vi "SingleElementsArray To Data_csm.vi"(7 "Pototype":variant, 8 "error in (no error)":errorcluster, 11 "DataElementArray":variant[](array[variant])) -> (0 "error out":errorcluster, 3 "Cluster":variant)   [LabVIEW 2017, in "API String Arguments Support.lvlib"]
doc: "This VI converts a DataELementArray to a Cluster."
uses:
  API String Arguments Support.lvlib
  <userlib>/_NEVSTOP/Communicable State Machine(CSM)/Communicable State Machine.lvlib
  <vilib>/Utility/Data Type/NI_Data Type.lvlib
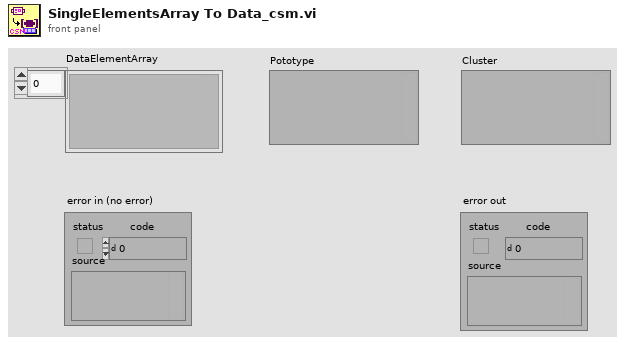
[diagram p1: front panel]
types:
  T1 = enum8{"<Null>", "I8", "I16", "I32", "I64", "U8", "U16", "U32", "U64", "SGL", "DBL", "EXT", "CSG", "CDB", "CXT", "0x0F", "0x10", "0x11", "0x12", "0x13", "0x14", "Enum U8", "Enum U16", "Enum U32", "Enum U64", "SGL PQ", "DBL PQ", "EXT PQ", "CSG PQ", "CDB PQ", "CXT PQ", "0x1F", "0x20", "Boolean", "0x22", "0x23", "0x24", "0x25", "0x26", "0x27", "0x28", "0x29", "0x2A", "0x2B", "0x2C", "0x2D", "0x2E", "0x2F", "String", "0x31", "Path", "Pict", "0x34", "0x35", "0x36", "DAQ", "0x38", "0x39", "0x3A", "0x3B", "0x3C", "0x3D", "0x3E", "0x3F", "Array", "0x41", "0x42", "0x43", "0x44", "0x45", "0x46", "0x47", "0x48", "0x49", "0x4A", "0x4B", "0x4C", "0x4D", "0x4E", "0x4F", "Cluster", "0x51", "0x52", "Variant", "Waveform", "0x55", "0x56", "0x57", "0x58", "0x59", "0x5A", "0x5B", "0x5C", "0x5D", "0x5E", "Fixed Point", "0x60", "0x61", "0x62", "0x63", "0x64", "0x65", "0x66", "0x67", "0x68", "0x69", "0x6A", "0x6B", "0x6C", "0x6D", "0x6E", "0x6F", "Refnum", "0x71", "0x72", "Set Collection", "Map Collection"}
  T2 = typedef "NI_Data Type.lvlib/Data Type.ctl" = enum8{"Invalid Type", "Void", "I8", "I16", "I32", "I64", "U8", "U16", "U32", "U64", "Single Float", "Double Float", "Extended Float", "Single Complex", "Double Complex", "Extended Complex", "Enum U8", "Enum U16", "Enum U32", "Enum U64", "Single Float With Unit", "Double Float With Unit", "Extended Float With Unit", "Single Complex with Unit", "Double Complex with Unit", "Extended Complex with Unit", "Boolean", "String", "Path", "Picture", "Tag", "Array", "Cluster", "Variant", "LV Variant", "Waveform", "Timestamp", "Digital Waveform", "Digital Data", "ExpressData", "Refnum", "External Data", "VI", "Poly VI", "LabVIEW Class Instance", "Fixed Point"}
  T3 = cluster{"length":u16, "private":u8, "type":enum8{"<Null>", "I8", "I16", "I32", "I64", "U8", "U16", "U32", "U64", "SGL", "DBL", "EXT", "CSG", "CDB", "CXT", "0x0F", "0x10", "0x11", "0x12", "0x13", "0x14", "Enum U8", "Enum U16", "Enum U32", "Enum U64", "SGL PQ", "DBL PQ", "EXT PQ", "CSG PQ", "CDB PQ", "CXT PQ", "0x1F", "0x20", "Boolean", "0x22", "0x23", "0x24", "0x25", "0x26", "0x27", "0x28", "0x29", "0x2A", "0x2B", "0x2C", "0x2D", "0x2E", "0x2F", "String", "0x31", "Path", "Pict", "0x34", "0x35", "0x36", "DAQ", "0x38", "0x39", "0x3A", "0x3B", "0x3C", "0x3D", "0x3E", "0x3F", "Array", "0x41", "0x42", "0x43", "0x44", "0x45", "0x46", "0x47", "0x48", "0x49", "0x4A", "0x4B", "0x4C", "0x4D", "0x4E", "0x4F", "Cluster", "0x51", "0x52", "Variant", "Waveform", "0x55", "0x56", "0x57", "0x58", "0x59", "0x5A", "0x5B", "0x5C", "0x5D", "0x5E", "Fixed Point", "0x60", "0x61", "0x62", "0x63", "0x64", "0x65", "0x66", "0x67", "0x68", "0x69", "0x6A", "0x6B", "0x6C", "0x6D", "0x6E", "0x6F", "Refnum", "0x71", "0x72", "Set Collection", "Map Collection"}, "# elements":u16}
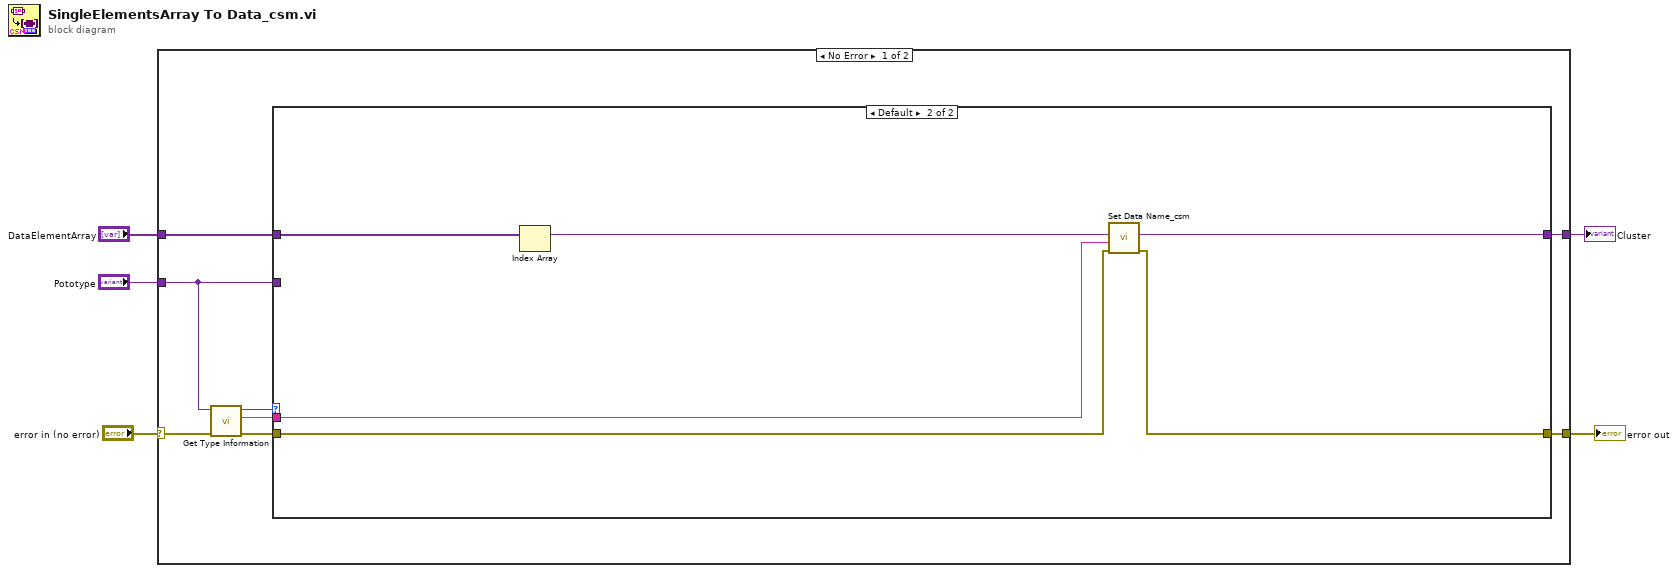
[diagram p0: block diagram]
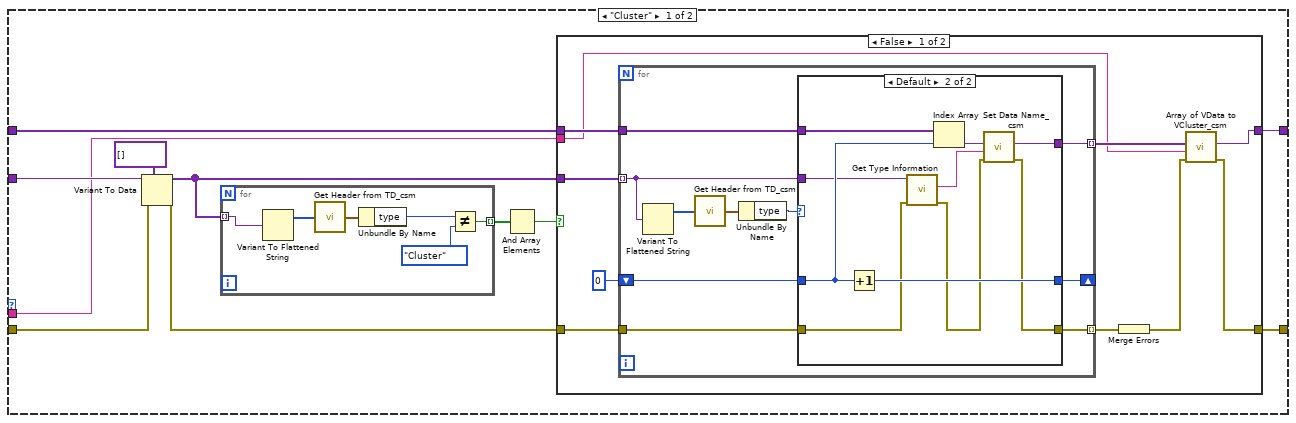
[diagram p2: hidden frame]
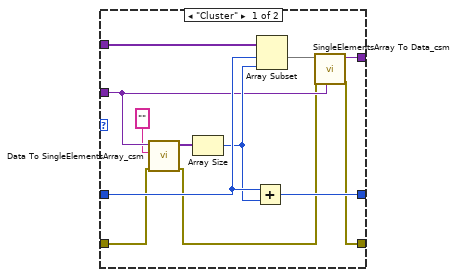
[diagram p3: hidden frame]
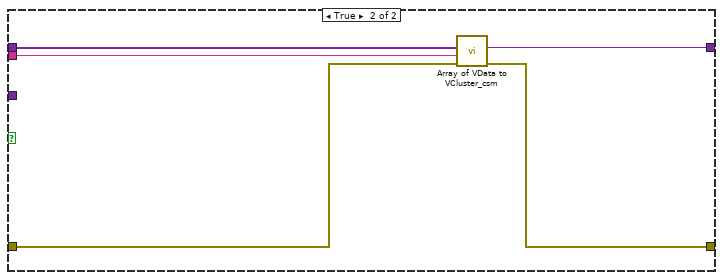
[diagram p4: hidden frame]
diagram:
  n1 = case shown="No Error" "error in (no error)" {
    selector: "error in (no error)" -> [w11 w84]
    tunnel: "DataElementArray" -> [w13 _]
    tunnel: [w12 w85] -> w4
    tunnel: [w10 w84] -> w2
    tunnel: "Pototype" -> [w8 w85]
    frame No Error {
      n2 = call <vilib>:"Get Type Information.vi"("error in (no error)"=w11, "Variant"=w8) -> ("error out"=w9:errorcluster, "Name"=w6:string, "Type"=w7:T2)  [unwired: 5 in, 2 out]
      n3 = case shown="Default" w7 {
        tunnel: w8 -> [w16 _]
        tunnel: w13 -> [w22 w83]
        tunnel: [w21 w81] -> w12
        tunnel: w9 -> [w15 w79]
        tunnel: [w20 w80] -> w10
        tunnel: w6 -> [w14 w78]
        frame "Cluster" {
          n4 = Variant To Data(error in=w15, type=variant[] [] ("Array"), Variant=w16) -> (data=w18:variant[], error out=w17:errorcluster)
          n5 = for {
            tunnel: w18 -> [w72] mode=indexing
            tunnel: [w76] -> w24 mode=indexing
            n6 = Variant To Flattened String(Variant=w72) -> (1:w75:i16[])  [unwired: 1 out]
            n7 = call <userlib>:"Get Header from TD_csm.vi"("Type Descriptor"=w75) -> ("Type Descriptor Header"=w74:T3)
            n8 = Unbundle By Name(w74) -> ("type"=w73:T1)
            n9 = Not Equal?(x=w73, y=T1."Cluster") -> (x != y?=w76:bool)
          }
          n10 = And Array Elements(Boolean array=w24) -> (logical AND=w23:bool)
          n11 = case shown="False" w23 {
            tunnel: w22 -> [w30 w71]
            tunnel: [w33 w70] -> w21
            tunnel: w18 -> [w34 _]
            tunnel: w17 -> [w29 w69]
            tunnel: [w25 w68] -> w20
            tunnel: w14 -> [w27 w67]
            frame False {
              n12 = for {
                tunnel: w34 -> [w36] mode=indexing
                tunnel: [w44] -> w32 mode=indexing
                shift-right: [w41] -> _
                shift-left: 0 -> [w42]
                tunnel: w30 -> [w43]
                tunnel: w29 -> [w40]
                tunnel: [w39] -> w28 mode=indexing
                n13 = Variant To Flattened String(Variant=w36) -> (1:w38:i16[])  [unwired: 1 out]
                n14 = call <userlib>:"Get Header from TD_csm.vi"("Type Descriptor"=w38) -> ("Type Descriptor Header"=w37:T3)
                n15 = Unbundle By Name(w37) -> ("type"=w35:T1)
                n16 = case shown="Default" w35 {
                  tunnel: w36 -> [w50 w59]
                  tunnel: [w56 w60] -> w44
                  tunnel: w43 -> [w55 w66]
                  tunnel: w42 -> [w54 w65]
                  tunnel: [w52 w64] -> w41
                  tunnel: w40 -> [w47 w58]
                  tunnel: [w45 w57] -> w39
                  frame "Cluster" {
                    n17 = call "Data To SingleElementsArray_csm.vi"("error in (no error)"=w47, "parentUrl"="", "Cluster"=w50) -> ("error out"=w46:errorcluster, "DataElementArray"=w48:variant[])  [unwired: 6 in, 1 out]
                    n18 = Array Size(array=w48) -> (size(s)=w53:i32)
                    n19 = Add(x=w54, y=w53) -> (x+y=w52:i32)
                    n20 = Array Subset(array=w55, index=w54, length=w53) -> (w51:variant[])
                    n21 = call "SingleElementsArray To Data_csm.vi"("Pototype"=w50, "error in (no error)"=w46, "DataElementArray"=w51) -> ("error out"=w45:errorcluster, "Cluster"=w56:variant)  [unwired: 7 in]
                  }
                  frame Default {
                    n22 = Increment(x=w65) -> (x+1=w64:i32)
                    n23 = call <vilib>:"Get Type Information.vi"("error in (no error)"=w58, "Variant"=w59) -> ("error out"=w62:errorcluster, "Name"=w63:string)  [unwired: 5 in, 3 out]
                    n24 = Index Array(array=w66, index=w65) -> (element=w61:variant)
                    n25 = call <userlib>:"Set Data Name_csm.vi"("error in (no error)"=w62, "Data Name"=w63, "Data"=w61) -> ("error out"=w57:errorcluster, "Renamed Data"=w60:variant)  [unwired: 7 in]
                  }
                }
              }
              n26 = Merge Errors(w28) -> (w26:errorcluster)
              n27 = call <userlib>:"Array of VData to VCluster_csm.vi"("error in (no error)"=w26, "Cluster Name"=w27, "Array"=w32) -> ("error out"=w25:errorcluster, "VCluster"=w33:variant)  [unwired: 7 in]
            }
            frame True {
              n28 = call <userlib>:"Array of VData to VCluster_csm.vi"("error in (no error)"=w69, "Cluster Name"=w67, "Array"=w71) -> ("error out"=w68:errorcluster, "VCluster"=w70:variant)  [unwired: 7 in]
            }
          }
        }
        frame Default {
          n29 = Index Array(array=w83) -> (element=w82:variant)  [unwired: 1 in]
          n30 = call <userlib>:"Set Data Name_csm.vi"("error in (no error)"=w79, "Data Name"=w78, "Data"=w82) -> ("error out"=w80:errorcluster, "Renamed Data"=w81:variant)  [unwired: 7 in]
        }
      }
    }
    frame Error {
    }
  }
  "error out" <- w2
  "Cluster" <- w4
